vi "Construct Delta JSON.vi"(9 "Force":bool, 10 "Checked Items":bool[](array[boolean]), 11 "JSON string":string) -> (3 "Delta JSON":string)   [LabVIEW 2019]
uses:
  <vilib>/MultiError/TokenizeJSON/Multi Error Cluster.lvlib
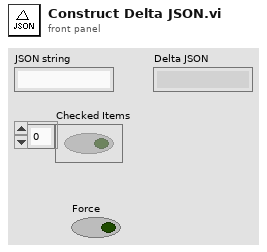
[diagram p1: front panel]
types:
  T1 = typedef "Multi Error Cluster.lvlib/JSON Token Descriptor.ctl" = cluster{"match string":string, "raw token type":T2, "byte offset ":i32}
  T2 = typedef "Multi Error Cluster.lvlib/JSON Raw Token Values.ctl" = enum32{"{", "}", "[", "]", ",", ":", "\"", "number", "string", "true", "false", "null", "invalid"}
  T3 = typedef "Multi Error Cluster.lvlib/JSON Token Values.ctl" = enum32{"array begin", "array end", "object begin", "object end", "value", "invalid", "name"}
  T4 = cluster{"whole match":string, "token index":i32}[]
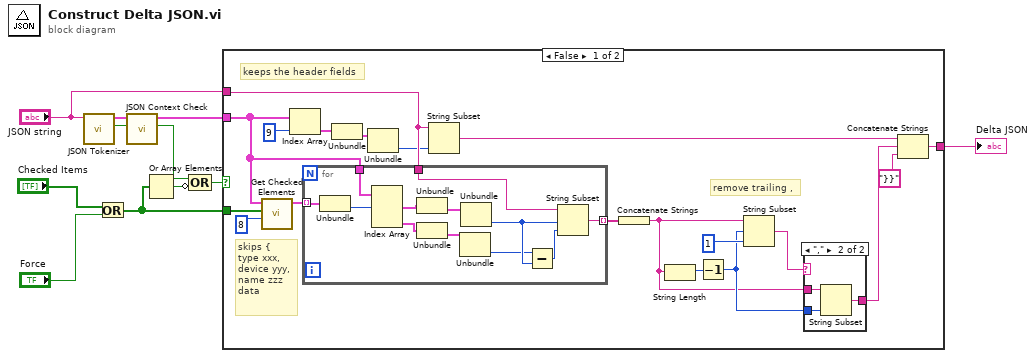
[diagram p0: block diagram]
diagram:
  n1 = call <vilib>:"JSON Tokenizer.vi"("JSON String"="JSON string") -> ("Invalid"=w11:bool, "Array"=w10:T1[])  [unwired: 9 in]
  n2 = Or(x="Checked Items", y="Force") -> (x .or. y?=w1:bool[])
  n3 = call <vilib>:"JSON Context Check.vi"("Invalid in"=w11, "Parse Tokens in"=w10) -> ("Invalid out"=w7:bool, "tokens"=w9:cluster{"token type":T3, "Type Definition":T1}[])  [unwired: 8 in]
  n4 = Or Array Elements(Boolean array=w1) -> (logical OR=w8:bool)
  n5 = Compound Arithmetic op=OR(w7, invert w8) -> (w6:bool)
  n6 = case shown="False" w6 {
    tunnel: w9 -> [w22 _]
    tunnel: w1 -> [w30 _]
    tunnel: "JSON string" -> [w21 _]
    tunnel: [w18 _] -> w4
    frame False {
      # "remove trailing ,"
      # "keeps the header fields"
      # "skips {\ntype xxx,\ndevice yyy,\nname zzz\ndata"
      n7 = call "Get Checked Elements.vi"("index"=8, "Checks"=w30, "tokens"=w22) -> ("Found Token Info"=w23:T4)  [unwired: 8 in]
      n8 = Index Array(array=w22, index=9) -> (element=w27:cluster{"token type":T3, "Type Definition":T1})
      n9 = for {
        tunnel: w23 -> [w42] mode=indexing
        tunnel: w22 -> [w41]
        tunnel: w21 -> [w37]
        tunnel: [w31] -> w20 mode=indexing
        n10 = Unbundle(w42) -> ("token index"=w40:i32)  [unwired: 1 out]
        n11 = Index Array(array=w41, index #1=w40) -> (element #1=w39:cluster{"token type":T3, "Type Definition":T1}, element #3=w36:cluster{"token type":T3, "Type Definition":T1})  [unwired: 2 in, 1 out]
        n12 = Unbundle(w39) -> ("Type Definition"=w38:T1)  [unwired: 1 out]
        n13 = Unbundle(w36) -> ("Type Definition"=w35:T1)  [unwired: 1 out]
        n14 = Unbundle(w35) -> ("byte offset"=w32:i32)  [unwired: 2 out]
        n15 = Unbundle(w38) -> ("byte offset"=w34:i32)  [unwired: 2 out]
        n16 = Subtract(x=w32, y=w34) -> (x-y=w33:i32)
        n17 = String Subset(string=w37, offset (0)=w34, length (rest)=w33) -> (substring=w31:string)
      }
      n18 = Unbundle(w27) -> ("Type Definition"=w26:T1)  [unwired: 1 out]
      n19 = Unbundle(w26) -> ("byte offset"=w17:i32)  [unwired: 2 out]
      n20 = String Subset(string=w21, length (rest)=w17) -> (substring=w25:string)  [unwired: 1 in]
      n21 = Concatenate Strings(w20) -> (w14:string)
      n22 = String Length(string=w14) -> (length=w19:i32)
      n23 = Decrement(x=w19) -> (x-1=w15:i32)
      n24 = String Subset(string=w14, offset (0)=w15, length (rest)=1 ("index")) -> (substring=w13:string)
      n25 = case shown="\",\"" w13 {
        tunnel: w15 -> [_ w44]
        tunnel: w14 -> [w43 w46]
        tunnel: [w43 w45] -> w12
        frame Default {
        }
        frame "," {
          n26 = String Subset(string=w46, length (rest)=w44) -> (substring=w45:string)  [unwired: 1 in]
        }
      }
      n27 = Concatenate Strings(w25, w12, "}}") -> (w18:string)
    }
    frame True {
    }
  }
  "Delta JSON" <- w4
